vi "input-cluster-data-to-file.vi"(0 "refnum in":refnum<file>, 3 "error in":errorcluster, 4 "Input - Cluster":T1 {"Dosiergeschw. [l/min]" format="%.2g"; "Dosiermenge [l]" format="%.1g"; "Füllstand  P" max=100 step=1 format="%#_3g"; "P-4 Drehzahl [%]" max=100 step=1 format="%#_3g"; "V-15 [%]" max=100 step=1 format="%_1g"; "V-13 [%]" max=100 step=1 format="%_1g"}) -> (7 "refnum out":refnum<file>, 10 "error out":errorcluster)   [LabVIEW 2011]
uses:
  Input - Cluster b2g2.ctl
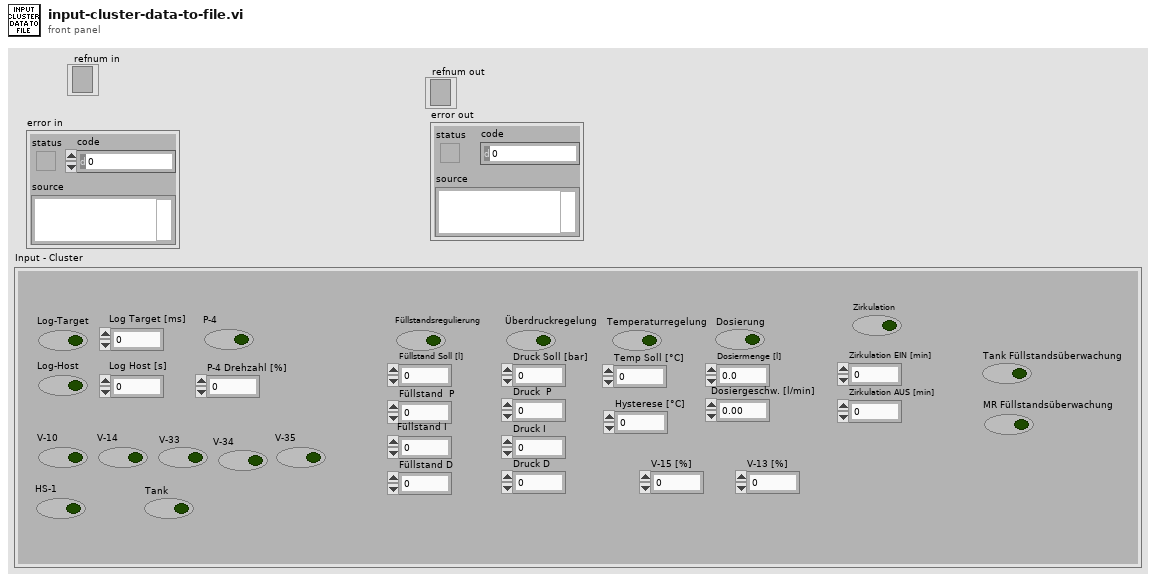
[diagram p1: front panel]
types:
  T1 = typedef "Input - Cluster b2g2.ctl" = cluster{"V-13 [%]":u8, "V-15 [%]":u8, "Log-Target":bool, "P-4":bool, "P-4 Drehzahl [%]":u8, "Temperaturregelung":bool, "Überdruckregelung":bool, "Füllstandsregulierung":bool, "V-10":bool, "Log-Host":bool, "V-14":bool, "HS-1":bool, "Füllstand  P":sgl, "Füllstand I":sgl, "Füllstand D":sgl, "Füllstand Soll [l]":sgl, "Druck  P":sgl, "Druck I":sgl, "Druck D":sgl, "Druck Soll [bar]":sgl, "Temp Soll [°C]":sgl, "Dosierung":bool, "Dosiermenge [l]":sgl, "Dosiergeschw. [l/min]":sgl, "Tank":bool, "Hysterese [°C]":sgl, "MR Füllstandsüberwachung":bool, "Tank Füllstandsüberwachung":bool, "Log Target [ms]":u32, "Log Host [s]":u32, "Zirkulation EIN [min]":u8, "Zirkulation AUS [min]":u8, "Zirkulation":bool, "V-33":bool, "V-34":bool, "V-35":bool}
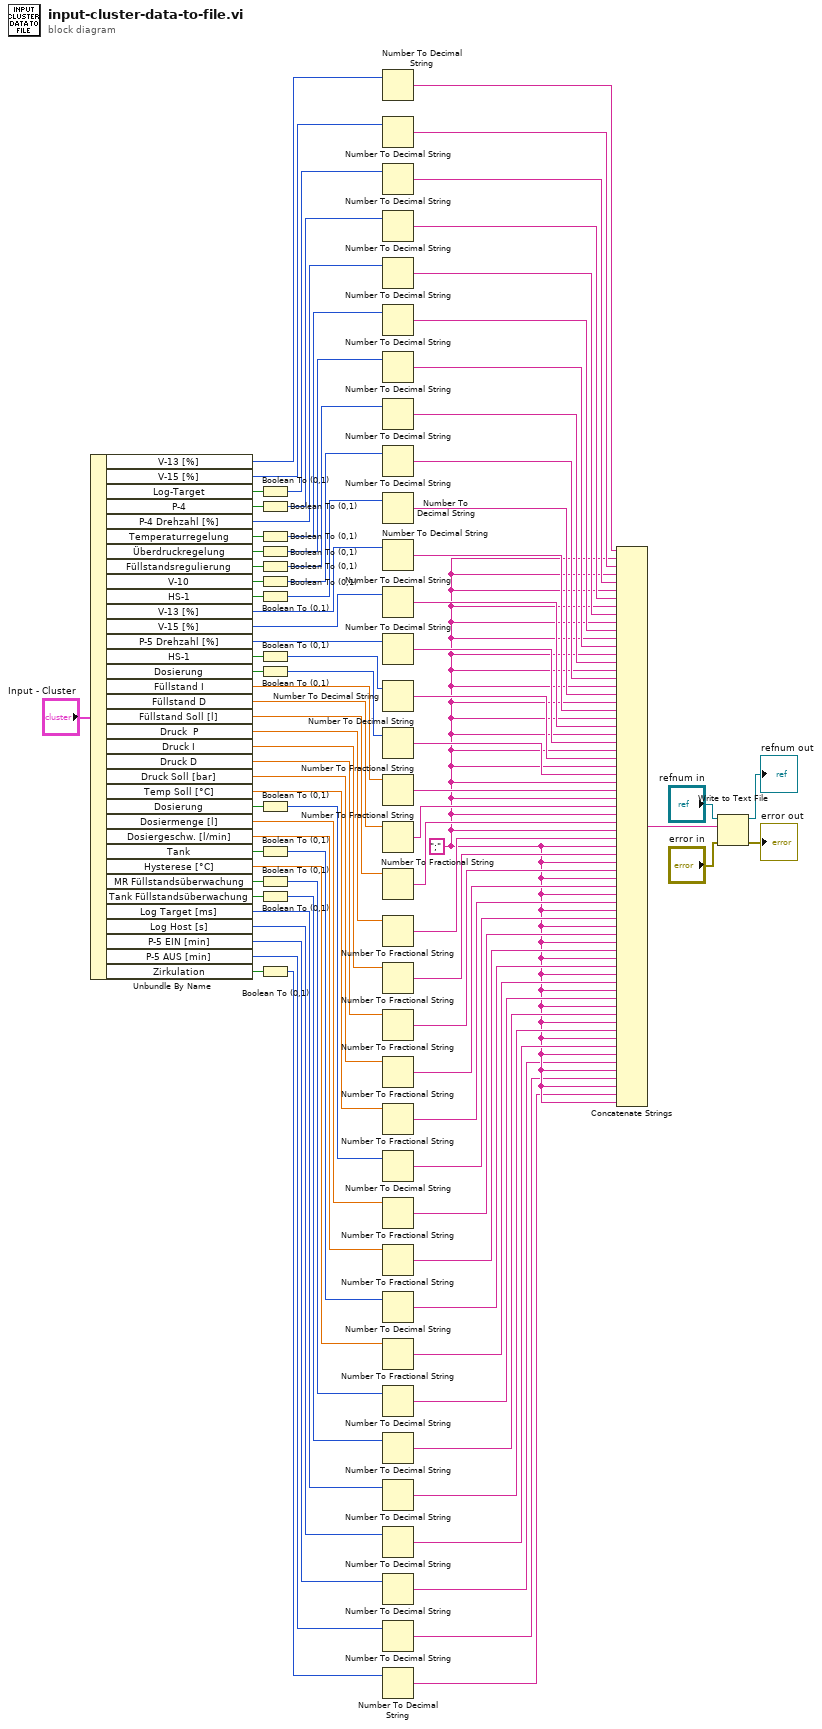
[diagram p0: block diagram]
diagram:
  w4 = ";" ("text")
  n1 = Unbundle By Name("Input - Cluster") -> ("V-13 [%]"=w80:u8, "V-15 [%]"=w53:u8, "Log-Target"=w62:bool, "P-4"=w61:bool, "P-4 Drehzahl [%]"=w50:u8, "Temperaturregelung"=w79:bool, "Überdruckregelung"=w60:bool, "Füllstandsregulierung"=w59:bool, "V-10"=w58:bool, "HS-1"=w78:bool, "V-13 [%]"=w73:u8, "V-15 [%]"=w72:u8, "P-5 Drehzahl [%]"=w71:u8, "HS-1"=w57:bool, "Dosierung"=w77:bool, "Füllstand I"=w45:sgl, "Füllstand D"=w44:sgl, "Füllstand Soll [l]"=w64:sgl, "Druck  P"=w43:sgl, "Druck I"=w42:sgl, "Druck D"=w41:sgl, "Druck Soll [bar]"=w40:sgl, "Temp Soll [°C]"=w39:sgl, "Dosierung"=w76:bool, "Dosiermenge [l]"=w37:sgl, "Dosiergeschw. [l/min]"=w36:sgl, "Tank"=w54:bool, "Hysterese [°C]"=w34:sgl, "MR Füllstandsüberwachung"=w56:bool, "Tank Füllstandsüberwachung"=w55:bool, "Log Target [ms]"=w10:u32, "Log Host [s]"=w9:u32, "P-5 EIN [min]"=w8:u8, "P-5 AUS [min]"=w7:u8, "Zirkulation"=w6:bool)
  n2 = Boolean To (0,1)(Boolean=w62) -> (0, 1=w52:i16)
  n3 = Boolean To (0,1)(Boolean=w61) -> (0, 1=w51:i16)
  n4 = Boolean To (0,1)(Boolean=w79) -> (0, 1=w75:i16)
  n5 = Boolean To (0,1)(Boolean=w60) -> (0, 1=w49:i16)
  n6 = Boolean To (0,1)(Boolean=w59) -> (0, 1=w48:i16)
  n7 = Boolean To (0,1)(Boolean=w58) -> (0, 1=w47:i16)
  n8 = Boolean To (0,1)(Boolean=w78) -> (0, 1=w74:i16)
  n9 = Boolean To (0,1)(Boolean=w57) -> (0, 1=w46:i16)
  n10 = Boolean To (0,1)(Boolean=w77) -> (0, 1=w70:i16)
  n11 = Boolean To (0,1)(Boolean=w76) -> (0, 1=w38:i16)
  n12 = Boolean To (0,1)(Boolean=w54) -> (0, 1=w35:i16)
  n13 = Boolean To (0,1)(Boolean=w56) -> (0, 1=w33:i16)
  n14 = Boolean To (0,1)(Boolean=w55) -> (0, 1=w32:i16)
  n15 = Boolean To (0,1)(Boolean=w6) -> (0, 1=w5:i16)
  n16 = Number To Decimal String(number=w80) -> (decimal integer string=w91:string)  [unwired: 1 in]
  n17 = Number To Decimal String(number=w53) -> (decimal integer string=w31:string)  [unwired: 1 in]
  n18 = Number To Decimal String(number=w52) -> (decimal integer string=w30:string)  [unwired: 1 in]
  n19 = Number To Decimal String(number=w51) -> (decimal integer string=w29:string)  [unwired: 1 in]
  n20 = Number To Decimal String(number=w50) -> (decimal integer string=w90:string)  [unwired: 1 in]
  n21 = Number To Decimal String(number=w75) -> (decimal integer string=w89:string)  [unwired: 1 in]
  n22 = Number To Decimal String(number=w49) -> (decimal integer string=w28:string)  [unwired: 1 in]
  n23 = Number To Decimal String(number=w48) -> (decimal integer string=w27:string)  [unwired: 1 in]
  n24 = Number To Decimal String(number=w47) -> (decimal integer string=w26:string)  [unwired: 1 in]
  n25 = Number To Decimal String(number=w74) -> (decimal integer string=w88:string)  [unwired: 1 in]
  n26 = Number To Decimal String(number=w73) -> (decimal integer string=w87:string)  [unwired: 1 in]
  n27 = Number To Decimal String(number=w72) -> (decimal integer string=w86:string)  [unwired: 1 in]
  n28 = Number To Decimal String(number=w71) -> (decimal integer string=w85:string)  [unwired: 1 in]
  n29 = Number To Decimal String(number=w46) -> (decimal integer string=w84:string)  [unwired: 1 in]
  n30 = Number To Decimal String(number=w70) -> (decimal integer string=w83:string)  [unwired: 1 in]
  n31 = Number To Fractional String(number=w45) -> (F-format string=w25:string)  [unwired: 3 in]
  n32 = Number To Fractional String(number=w44) -> (F-format string=w24:string)  [unwired: 3 in]
  n33 = Number To Fractional String(number=w64) -> (F-format string=w65:string)  [unwired: 3 in]
  n34 = Number To Fractional String(number=w43) -> (F-format string=w23:string)  [unwired: 3 in]
  n35 = Number To Fractional String(number=w42) -> (F-format string=w22:string)  [unwired: 3 in]
  n36 = Number To Fractional String(number=w41) -> (F-format string=w21:string)  [unwired: 3 in]
  n37 = Number To Fractional String(number=w40) -> (F-format string=w20:string)  [unwired: 3 in]
  n38 = Number To Fractional String(number=w39) -> (F-format string=w19:string)  [unwired: 3 in]
  n39 = Number To Decimal String(number=w38) -> (decimal integer string=w82:string)  [unwired: 1 in]
  n40 = Number To Fractional String(number=w37) -> (F-format string=w18:string)  [unwired: 3 in]
  n41 = Number To Fractional String(number=w36) -> (F-format string=w17:string)  [unwired: 3 in]
  n42 = Number To Decimal String(number=w35) -> (decimal integer string=w16:string)  [unwired: 1 in]
  n43 = Number To Fractional String(number=w34) -> (F-format string=w15:string)  [unwired: 3 in]
  n44 = Number To Decimal String(number=w33) -> (decimal integer string=w14:string)  [unwired: 1 in]
  n45 = Number To Decimal String(number=w32) -> (decimal integer string=w13:string)  [unwired: 1 in]
  n46 = Number To Decimal String(number=w10) -> (decimal integer string=w12:string)  [unwired: 1 in]
  n47 = Number To Decimal String(number=w9) -> (decimal integer string=w11:string)  [unwired: 1 in]
  n48 = Number To Decimal String(number=w8) -> (decimal integer string=w3:string)  [unwired: 1 in]
  n49 = Number To Decimal String(number=w7) -> (decimal integer string=w2:string)  [unwired: 1 in]
  n50 = Number To Decimal String(number=w5) -> (decimal integer string=w1:string)  [unwired: 1 in]
  n51 = Concatenate Strings(w91, w4, w31, w4, w30, w4, w29, w4, w90, w4, w89, w4, w28, w4, w27, w4, w26, w4, w88, w4, w87, w4, w86, w4, w85, w4, w84, w4, w83, w4, w25, w4, w24, w4, w65, w4, w23, w4, w22, w4, w21, w4, w20, w4, w19, w4, w82, w4, w18, w4, w17, w4, w16, w4, w15, w4, w14, w4, w13, w4, w12, w4, w11, w4, w3, w4, w2, w4, w1, w4) -> (w81:string)
  n52 = Write to Text File(file (use dialog)="refnum in", text=w81, error in="error in") -> (refnum out=→"refnum out":refnum<file>, error out=→"error out":errorcluster)  [unwired: 1 in, 1 out]
